vi "Rosie-Toggle-Output.vi"(8 "error in (no error)":errorcluster, 11 "connection ID":refnum<k5>) -> (0 "error out":errorcluster, 3 "connection ID out":refnum<k5>)   [LabVIEW 2020]
panel:
  # "Rosie Toggle Output"
  # "Toggles the secondary trigger output on or off."
  # "Input an already-opened TCP connection to a Rosie device."
  # "Concrete actions:\n1. Read current value of output.\n2. Set output to opposite value."
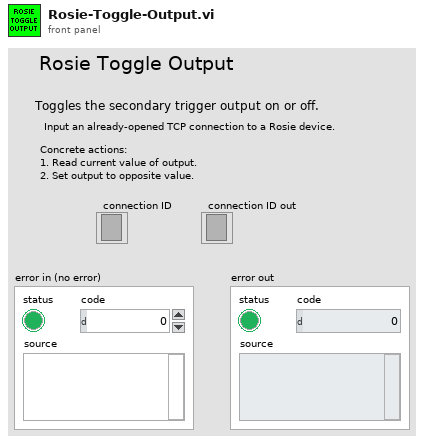
[diagram p1: front panel]
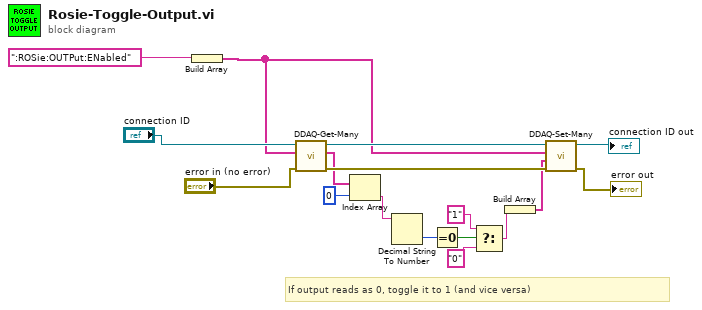
[diagram p0: block diagram]
diagram:
  # "If output reads as 0, toggle it to 1 (and vice versa)"
  n1 = Build Array(":ROSie:OUTPut:ENabled") -> (w8:string[])
  n2 = call "DDAQ-Get-Many.vi"("error in (no error)"="error in (no error)", "SCPI-like Keywords (leave off question marks)"=w8, "connection ID"="connection ID") -> ("error out"=w12:errorcluster, "Responses"=w11:string[], "connection ID out"=w14:refnum<k5>)  [unwired: 4 in, 2 out]
  n3 = Index Array(array=w11, index=0) -> (element=w7:string)
  n4 = Decimal String To Number(string=w7) -> (number=w6:i32)  [unwired: 2 in, 1 out]
  n5 = Equal To 0?(x=w6) -> (x = 0?=w5:bool)
  n6 = Select(t="1" ("Set Value"), s=w5, f="0" ("Set Value")) -> (s? t:f=w2:string)
  n7 = Build Array(w2) -> (w1:string[])
  n8 = call "DDAQ-Set-Many.vi"("error in (no error)"=w12, "Set Values"=w1, "SCPI-like Keywords (leave off space, value)"=w8, "connection ID"=w14) -> ("error out"=→"error out":errorcluster, "connection ID out"=→"connection ID out":refnum<k5>)  [unwired: 5 in, 1 out]
